vi "Sinus.vi"(1 "Phase phi":dbl(slide) scale=0.0..3.14159, 2 "Amplitude A":dbl(slide)=1.1111111111111112 scale=0.0..10.0, 3 "Frequenz f":dbl(slide)=10.101010101010102 scale=0.0..100.0, 4 "Datenpunkte N":i32(slide)=1000 scale=0.0..1000.0) -> (0 "sin(t_i)":dbl[](array[numeric]))   [LabVIEW 2017]
uses:
  <vilib>/express/express analysis/Spectral/Block/exnSpectralBlock spectral measurements power poly.vi
  <vilib>/express/express analysis/Spectral/Block/exnSpectralBlock spectral measurements power WFM.vi
  <vilib>/express/express analysis/Spectral/XNode/ExpressSpectralMeasurementsBlockNode.xnode
panel:
  out "Waveform Graph":cluster{"f0":dbl, "df":dbl, "magnitude":dbl[]}(graph)
  out "XY Graph 2":cluster{dbl[], dbl[]}(graph)
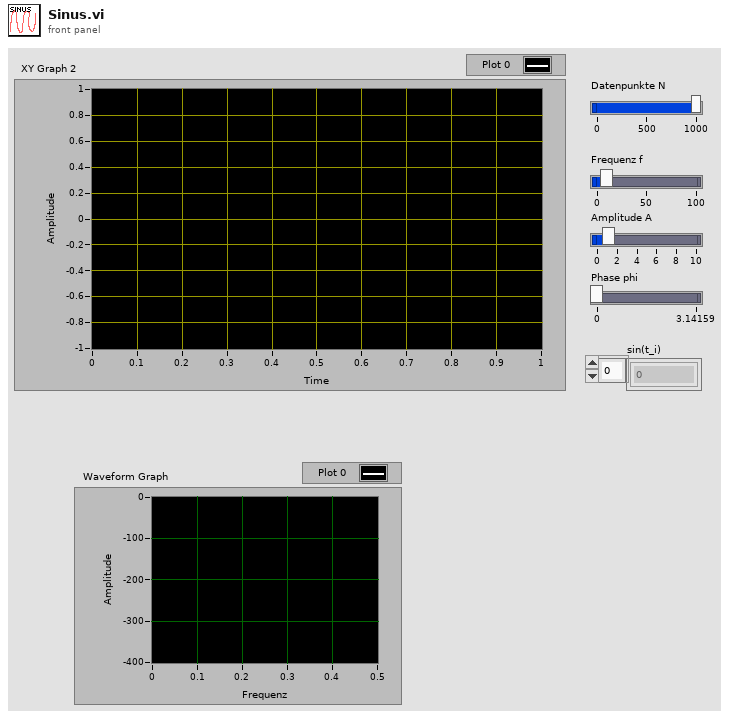
[diagram p1: front panel]
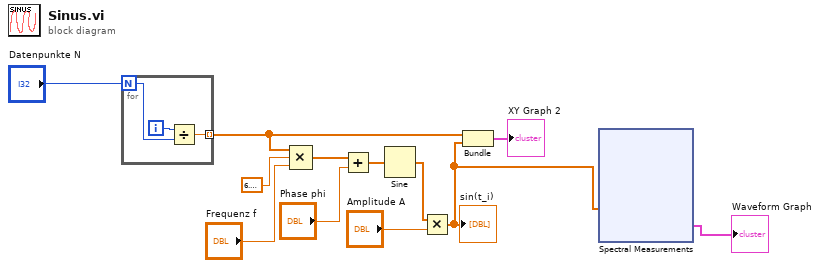
[diagram p0: block diagram]
diagram:
  n1 = for {
    N: "Datenpunkte N" -> [w15]
    tunnel: [w13] -> w4 mode=indexing
    i -> [w14]
    n2 = Divide(x=w14, y=w15) -> (x/y=w13:dbl)
  }
  n3 = Compound Arithmetic op=MULTIPLY(w4, 6.283185307179586, "Frequenz f") -> (w9:dbl[])
  n4 = Add(x=w9, y="Phase phi") -> (x+y=w8:dbl[])
  n5 = Sine(x=w8) -> (sin(x)=w7:dbl[])
  n6 = Multiply(x=w7, y="Amplitude A") -> (x*y=w2:dbl[])
  "sin(t_i)" <- w2
  n7 = Bundle(w4, w2) -> (→"XY Graph 2":cluster{dbl[], dbl[]})  [unwired: 1 in]
  n8 = xnode "Spectral Measurements"("Signals"=w2) -> ("Power Spectrum"=→"Waveform Graph":cluster{"f0":dbl, "df":dbl, "magnitude":dbl[]})  [unwired: 1 in, 1 out]
